vi "Serial Commands Engineering Tool.vi"() -> ()   [LabVIEW 2012]
uses:
  Type Defs/Named Final Output.ctl
  Type Defs/Data Reading.ctl
  <vilib>/Instr/_visa.llb/VISA Flush IO Buffer Mask.ctl
panel:
  in  "Warmup if ON":bool
  in  "Mask":T1=16 items=["Flush Receive Buffer"=16, "Write Transmit Buffer to Device"=32, "Flush Receive Buffer (No I/O)"=64, "Flush Transmit Buffer"=128]
  in  "Just Read":bool
  out "Cal Data":T2={"Time"="20:36:08", "Consecutive good readings"=4, "Total readings"=-1, "A/D counts Sensor 1"=3314.919, "A/D counts Sensor 2"=3314.935, "Diff current/previous Sensor 1"=-0.155, "Diff current/previous Sensor 2"=-0.099}
  out "Data Read":T3 {"Last Ctrl Word" format="%.0x"}
  in  "Other Outputs":cluster{"Alarm":bool, "Heater":bool}
  in  "Final Output Controls":T4
  in  "Start O2 Calibration 5-10 Minutes":bool
  in  "Check Firmware":bool
  in  "Read RT Clock":bool
  out "Current error":errorcluster
  in  "Set RT Clock":bool
  in  "CAT On/Off":bool=TRUE
  in  "Date string":string
  out "Version":string="\r\n"
  out "RT Clock":string
  in  "stop":bool
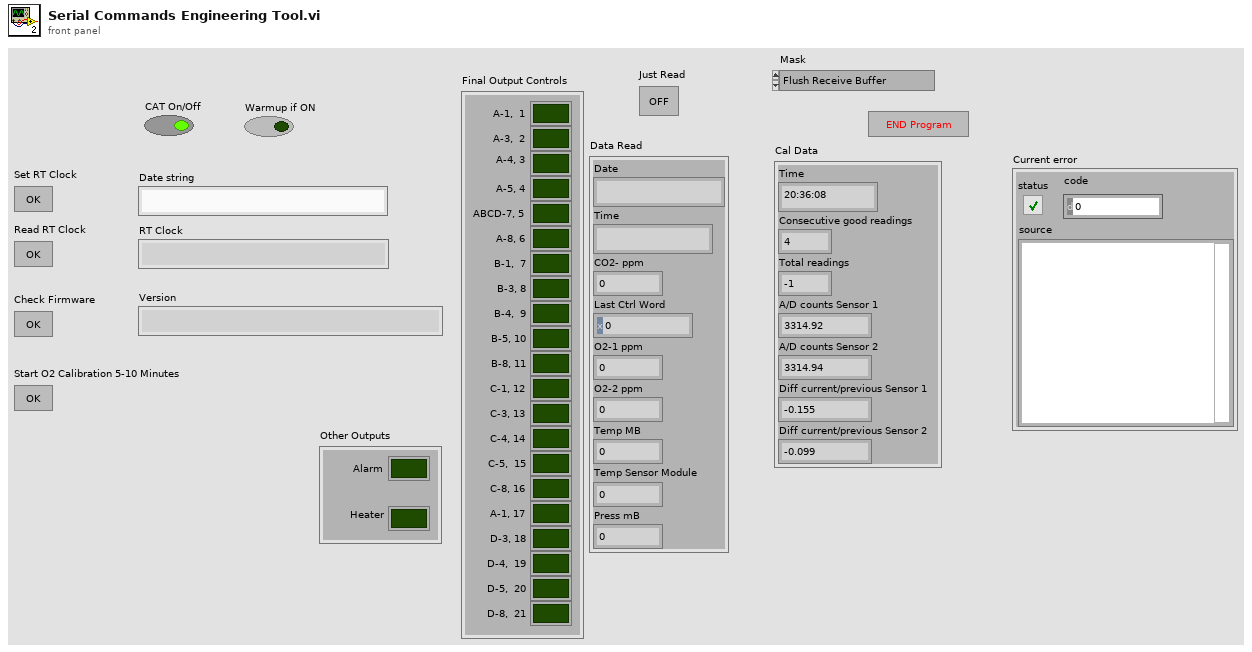
[diagram p1: front panel]
types:
  T1 = typedef "VISA Flush IO Buffer Mask.ctl" = u16
  T2 = cluster{"Time":string, "Consecutive good readings":i32, "Total readings":i32, "A/D counts Sensor 1":sgl, "A/D counts Sensor 2":sgl, "Diff current/previous Sensor 1":sgl, "Diff current/previous Sensor 2":sgl}
  T3 = typedef "Data Reading.ctl" = cluster{"Date":string, "Time":string, "CO2- ppm":u32, "Last Ctrl Word":u32, "O2-1 ppm":u32, "O2-2 ppm":u32, "Temp MB":sgl, "Temp Sensor Module":sgl, "Press mB":sgl}
  T4 = typedef "Named Final Output.ctl" = cluster{"A-1,  1":bool, "A-3,  2":bool, "A-4, 3":bool, "A-5, 4":bool, "ABCD-7, 5":bool, "A-8, 6":bool, "B-1,  7":bool, "B-3, 8":bool, "B-4,  9":bool, "B-5, 10":bool, "B-8, 11":bool, "C-1, 12":bool, "C-3, 13":bool, "C-4, 14":bool, "C-5,  15":bool, "C-8, 16":bool, "A-1, 17":bool, "D-3, 18":bool, "D-4,  19":bool, "D-5,  20":bool, "D-8,  21":bool}
  T5 = cluster{"Date":string, "Time":string, "CO2- ppm":u32, "Last Ctrl Word":u32, "O2-1 ppm":u32, "O2-2 ppm":u32, "Temp MB":sgl, "Temp Sensor Module":sgl, "Press mB":sgl}
  T6 = cluster{"Date":string, "Time":string, "CO2- ppm":u32, "Last Ctrl Word":u32, "O2-1 ppm":u32, "O2-2 ppm":u32, "Temp MB":sgl, "Temp Sensor Modulr":sgl, "Press mB":sgl}
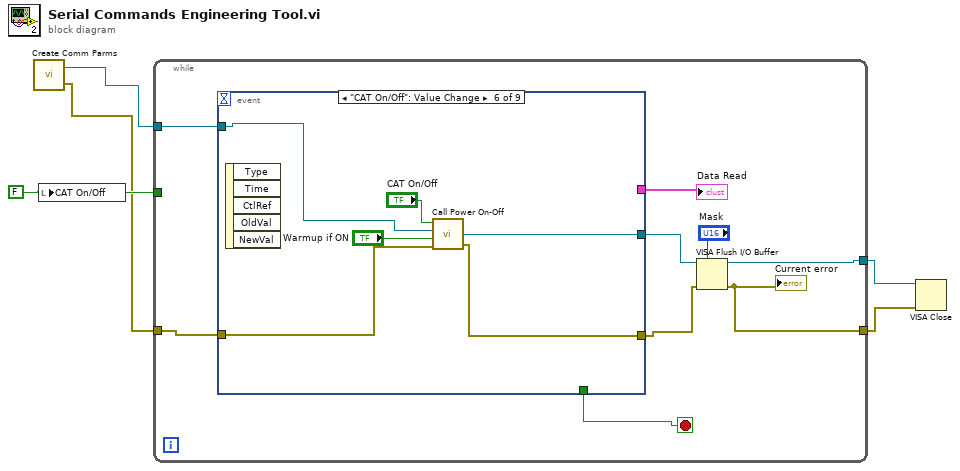
[diagram p0: block diagram]
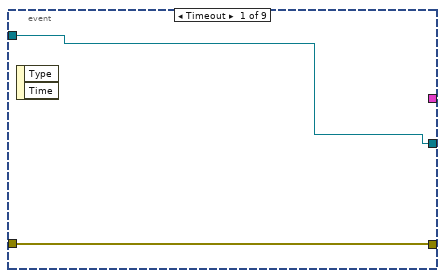
[diagram p2: hidden frame]
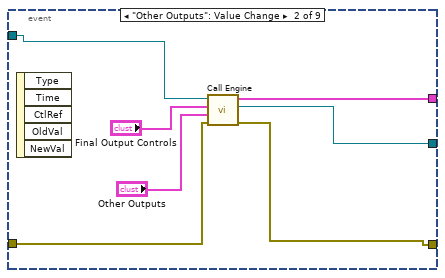
[diagram p3: hidden frame]
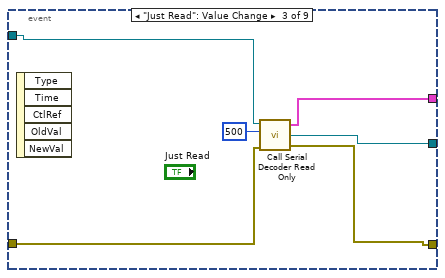
[diagram p4: hidden frame]
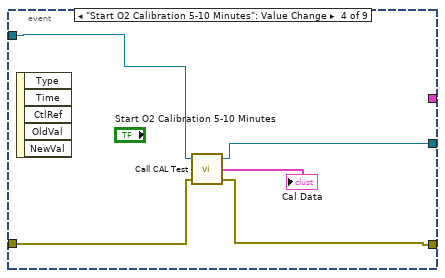
[diagram p5: hidden frame]
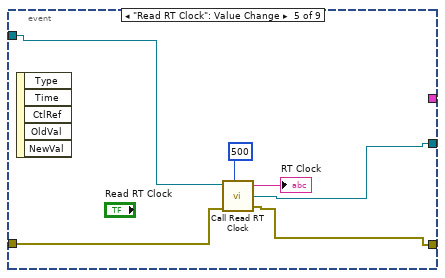
[diagram p6: hidden frame]
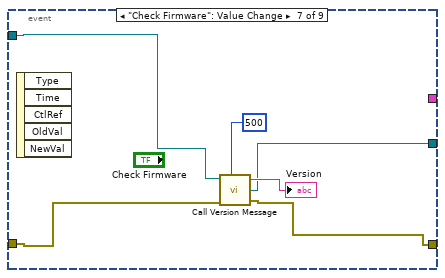
[diagram p7: hidden frame]
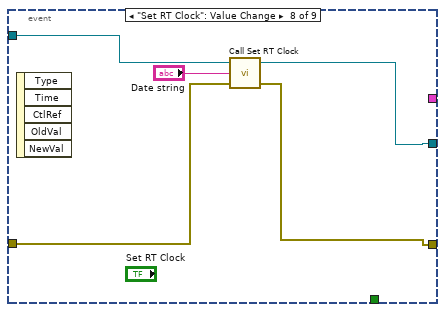
[diagram p8: hidden frame]
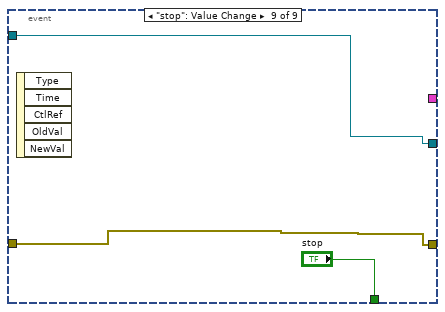
[diagram p9: hidden frame]
diagram:
  w5 = FALSE ("CAT On/Off")
  n1 = call "Create Comm Parms.vi"() -> ("error out"=w3:errorcluster, "VISA resource name out"=w4:refnum<visa-resource-name>)  [unwired: 2 in]
  n2 = local write "CAT On/Off"(w5) -> ()
  n3 = while {
    tunnel: w4 -> [w14]
    tunnel: w5 -> [_]
    tunnel: [w9] -> w1
    tunnel: w3 -> [w13]
    tunnel: [w7] -> w2
    stop <- w12 stop-if-true
    n4 = event shown="[5] \"CAT On/Off\": Value Change" {
      selector: _ -> [_ _ _ _ _ _ _ _ _]
      dyn-events: _ -> [_ _ _ _ _ _ _ _ _]
      timeout: _ -> [_ _ _ _ _ _ _ _ _]
      tunnel: w14 -> [w15 w17 w25 w31 w36 w43 w48 w54 w58]
      tunnel: w13 -> [w16 w21 w29 w34 w39 w45 w51 w56 w59]
      tunnel: [w16 w20 w28 w33 w38 w44 w50 w55 w59] -> w8
      tunnel: [_ _ _ _ _ _ _ _ "stop"] -> w12
      tunnel: [_ w19 w27 _ _ _ _ _ _] -> w11
      tunnel: [w15 w18 w24 w30 w35 w42 w47 w53 w58] -> w10
      event Timeout {
        n5 = event-data() -> ()  [unwired: 1 in, 2 out]
      }
      event "Other Outputs": Value Change {
        n6 = event-data() -> ()  [unwired: 1 in, 5 out]
        n7 = call "Call Engine.vi"("error in"=w21, "Other Outputs"="Other Outputs", "Final Output Controls"="Final Output Controls", "Port"=w17) -> ("error out"=w20:errorcluster, "VISA resource name out"=w18:refnum<visa-resource-name>, "Data Read"=w19:T5)  [unwired: 1 in, 1 out]
      }
      event "Just Read": Value Change {
        n8 = event-data() -> ()  [unwired: 1 in, 5 out]
        n9 = call "Call Serial Decoder Read Only.vi"("VISA resource name"=w25, "milliseconds to wait"=u32 500, "error in"=w29) -> ("Data Read"=w27:T6, "VISA resource name out"=w24:refnum<visa-resource-name>, "error out"=w28:errorcluster)  [unwired: 2 in]
      }
      event "Start O2 Calibration 5-10 Minutes": Value Change {
        n10 = event-data() -> ()  [unwired: 1 in, 5 out]
        n11 = call "Call CAL Test.vi"("error in (no error)"=w34, "VISA resource name"=w31) -> ("error out"=w33:errorcluster, "Cal Data"=→"Cal Data":T2, "VISA resource name out"=w30:refnum<visa-resource-name>)  [unwired: 1 in]
      }
      event "Read RT Clock": Value Change {
        n12 = event-data() -> ()  [unwired: 1 in, 5 out]
        n13 = call "Call Read RT Clock.vi"("VISA resource name out"=w36, "delay before read (ms)"=u32 500, "error in"=w39) -> ("read string"=→"RT Clock":string, "VISA resource name out 2"=w35:refnum<visa-resource-name>, "error out"=w38:errorcluster)  [unwired: 3 in]
      }
      event "CAT On/Off": Value Change {
        n14 = event-data() -> ()  [unwired: 1 in, 5 out]
        n15 = call "Call Power On-Off.vi"("error in"=w45, "Warmup if ON"="Warmup if ON", "VISA resource name"=w43, "On/Off"="CAT On/Off") -> ("error out"=w44:errorcluster, "VISA resource name out"=w42:refnum<visa-resource-name>)  [unwired: 1 in]
      }
      event "Check Firmware": Value Change {
        n16 = event-data() -> ()  [unwired: 1 in, 5 out]
        n17 = call "Call Version Message.vi"("VISA resource name out"=w48, "delay before read (ms)"=u32 500, "error in"=w51) -> ("read string"=→"Version":string, "VISA resource name out 2"=w47:refnum<visa-resource-name>, "error out"=w50:errorcluster)  [unwired: 2 in, 1 out]
      }
      event "Set RT Clock": Value Change {
        n18 = event-data() -> ()  [unwired: 1 in, 5 out]
        n19 = call "Call Set RT Clock.vi"("error in"=w56, "Date string"="Date string", "VISA resource name"=w54) -> ("error out"=w55:errorcluster, "VISA resource name out"=w53:refnum<visa-resource-name>)  [unwired: 1 in]
      }
      event "stop": Value Change {
        n20 = event-data() -> ()  [unwired: 1 in, 5 out]
      }
    }
    "Data Read" <- w11
    n21 = VISA Flush I/O Buffer(VISA resource name=w10, mask (16)="Mask", error in (no error)=w8) -> (VISA resource name out=w9:refnum<visa-resource-name>, error out=w7:errorcluster)
    "Current error" <- w7
  }
  n22 = VISA Close(VISA resource name=w1, error in (no error)=w2) -> ()  [unwired: 1 out]
